vi "Read_Motor_Load.vi"(8 "error in (no error)":errorcluster, 9 "Address":u8=40, 11 "VISA Refnum in":refnum<visa-resource-name>) -> (0 "error out":errorcluster, 2 "Current load":dbl, 3 "VISA Refnum out":refnum<visa-resource-name>)   [LabVIEW 2015]
uses:
  <instrlib>/Dynamixel Motor/Dynamixel Motor.lvlib
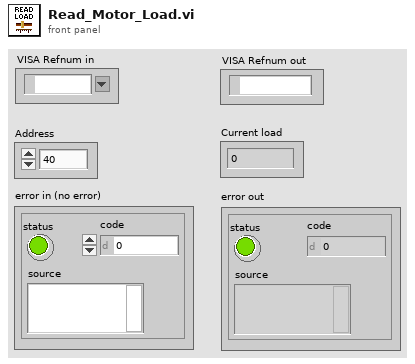
[diagram p1: front panel]
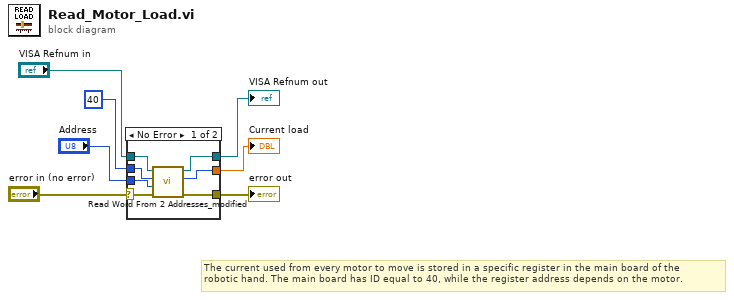
[diagram p0: block diagram]
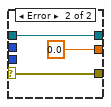
[diagram p2: hidden frame]
diagram:
  # "The current used from every motor to move is stored in a specific register in the main board of the \nrobotic hand. The main board has ID equal to 40, while the register address depends on the motor."
  n1 = case shown="No Error" "error in (no error)" {
    selector: "error in (no error)" -> [w11 w16]
    tunnel: "VISA Refnum in" -> [w14 w17]
    tunnel: [w10 w17] -> w2
    tunnel: [w8 w16] -> w7
    tunnel: [w9 0.0] -> w6
    tunnel: u8 40 ("Motor ID (0)") -> [w13 _]
    tunnel: "Address" -> [w12 _]
    frame No Error {
      n2 = call "Read Word From 2 Addresses_modified.vi"("Error in (no error)"=w11, "Address number (0)"=w12, "Motor ID (0)"=w13, "VISA resource name"=w14) -> ("error out"=w8:errorcluster, "Data"=w9:u16, "VISA resource name out"=w10:refnum<visa-resource-name>)  [unwired: 5 in]
    }
    frame Error {
    }
  }
  "error out" <- w7
  "Current load" <- w6
  "VISA Refnum out" <- w2
